vi "ITC 503 -- save sweep table.vi"(6 "Set Temperature":dbl, 7 "Sweep Table":dbl[][](array[numeric])=[[150.0, 1399.0, 0.0], [20.0, 1399.0, 0.0], [150.0, 1399.0, 0.0], [300.0, 1399.0, 0.0], [295.0, 10.0, 1399.0], [295.0, 10.0, 1399.0]], 8 "error in":errorcluster, 10 "Base Path":path, 11 "Base name":string="SweepTable_") -> (0 "error out":errorcluster, 3 "saving sweep table to":string="C:\\data\\RUS\\Experiment\\YBCO_4\\Sweep10\\SweepTable_061411.dat")   [LabVIEW 2010]
uses:
  <vilib>/Utility/file.llb/Write To Spreadsheet File (string).vi
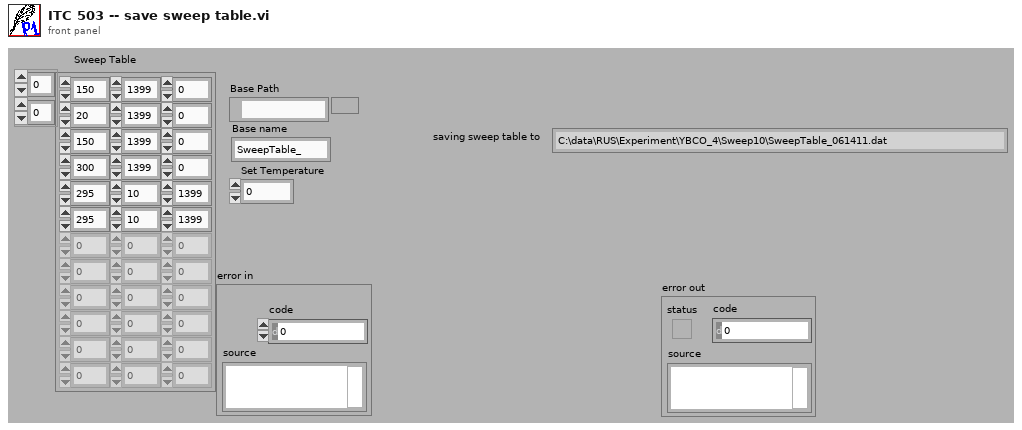
[diagram p1: front panel]
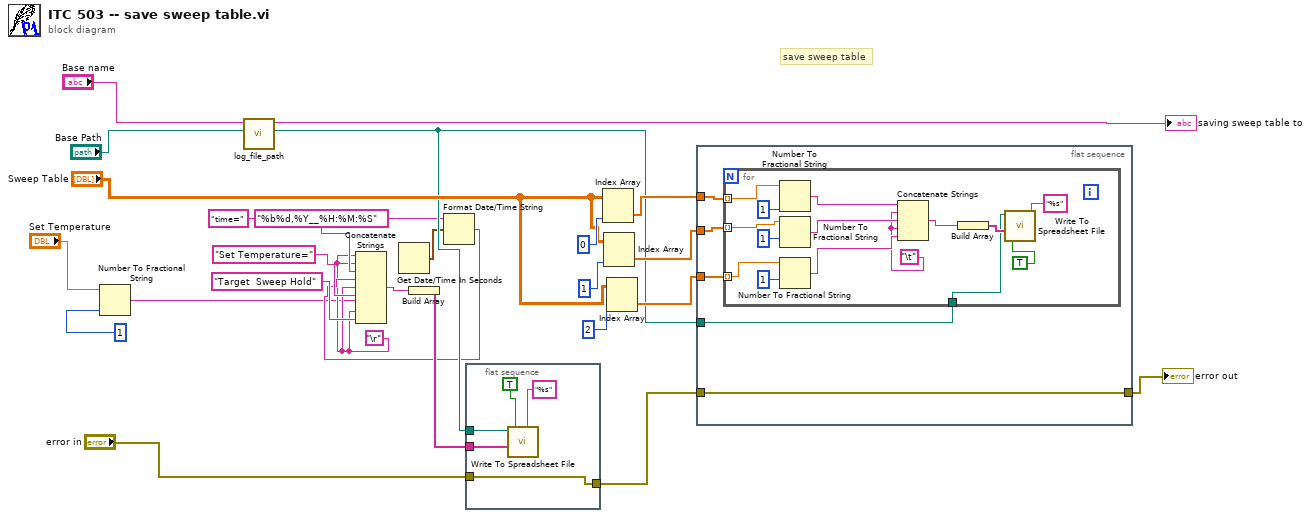
[diagram p0: block diagram]
diagram:
  w7 = "\r"
  # "save sweep table"
  n1 = Number To Fractional String(number="Set Temperature", precision (6)=i16 1) -> (F-format string=w1:string)  [unwired: 2 in]
  n2 = call "log_file_path.vi"("base path in"="Base Path", "base name in"="Base name") -> ("path out"=w16:path, "string path out"=→"saving sweep table to":string)  [unwired: 8 in]
  n3 = Get Date/Time In Seconds() -> (seconds since 1Jan1904=w11:timestamp)
  n4 = Format Date/Time String(time format string (%c)="%b%d,%Y__%H:%M:%S", seconds (now)=w11) -> (date/time string=w9:string)  [unwired: 1 in]
  n5 = Concatenate Strings(w7, w7, "time=" ("string"), w9, w7, "Set Temperature=" ("Command"), w1, w7, "Target  Sweep Hold" ("Command")) -> (w13:string)
  n6 = Build Array(w13) -> (w14:string[])
  n7 = flat-sequence {
    tunnel: w16 -> [w31]
    tunnel: w14 -> [w28]
    tunnel: [w27] -> w5
    tunnel: "error in" -> [w27]
    frame #0 {
      n8 = call-poly <vilib>:"Write To Spreadsheet File.vi"("format (%s)"="%s" ("format (%.3f)"), "append to file? (new file:F)"=TRUE, "1D data"=w28, "file path (dialog if empty)"=w31) -> ()  [unwired: 4 in, 1 out]
    }
  }
  n9 = Index Array(array="Sweep Table", index (col)=0 ("disabled index (col)")) -> (element=w24:dbl[])  [unwired: 1 in]
  n10 = Index Array(array="Sweep Table", index (col)=1 ("disabled index (col)")) -> (element=w25:dbl[])  [unwired: 1 in]
  n11 = Index Array(array="Sweep Table", index (col)=2 ("disabled index (col)")) -> (element=w26:dbl[])  [unwired: 1 in]
  n12 = flat-sequence {
    tunnel: w26 -> [w36]
    tunnel: w25 -> [w35]
    tunnel: w24 -> [w34]
    tunnel: w16 -> [w33]
    tunnel: [w32] -> w6
    tunnel: w5 -> [w32]
    frame #0 {
      n13 = for {
        tunnel: w34 -> [w50] mode=indexing
        tunnel: w35 -> [w48] mode=indexing
        tunnel: w36 -> [w46] mode=indexing
        tunnel: w33 -> [w37]
        w38 = "\t"
        n14 = Number To Fractional String(number=w50, precision (6)=i16 1) -> (F-format string=w45:string)  [unwired: 2 in]
        n15 = Number To Fractional String(number=w48, precision (6)=i16 1) -> (F-format string=w44:string)  [unwired: 2 in]
        n16 = Number To Fractional String(number=w46, precision (6)=i16 1) -> (F-format string=w43:string)  [unwired: 2 in]
        n17 = Concatenate Strings(w45, w38, w44, w38, w43) -> (w39:string)
        n18 = Build Array(w39) -> (w40:string[])
        n19 = call-poly <vilib>:"Write To Spreadsheet File.vi"("format (%s)"="%s" ("format (%.3f)"), "append to file? (new file:F)"=TRUE, "1D data"=w40, "file path (dialog if empty)"=w37) -> ()  [unwired: 4 in, 1 out]
      }
    }
  }
  "error out" <- w6
